vi "Log.vi"(0 "error handler in":refnum<class "TLB` Error Handler.lvclass">) -> (4 "error handler out":refnum<class "TLB` Error Handler.lvclass">, 15 "error out":errorcluster)   [LabVIEW 2015, in "TLB` Template.lvlib" / "TLB` Error Handler.lvclass"]
doc: "write capture errors to disk.\n\n<B>Input Parameters</B>\n\n<B>error handler in</B> dentifies your session. <B>Error Handler in</B> is obtained from the Open.vi of this class.\n\n<B>Output Parameters</B>\n\n<B>error handler out</B> identifies your session. <B>Error Handler out</B> is obtained from the Open.vi of this class.\n\n<B>error out</B> contains error information. This output provides standard error out functionality."
uses:
  TLB` Error Handler.lvclass
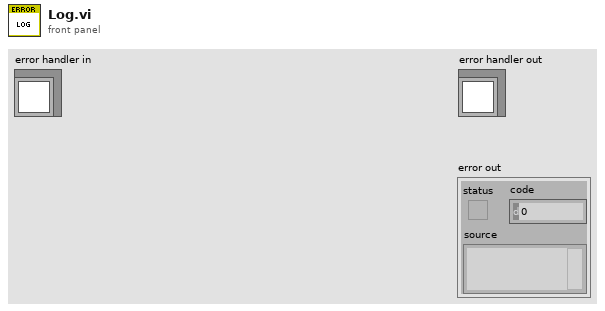
[diagram p1: front panel]
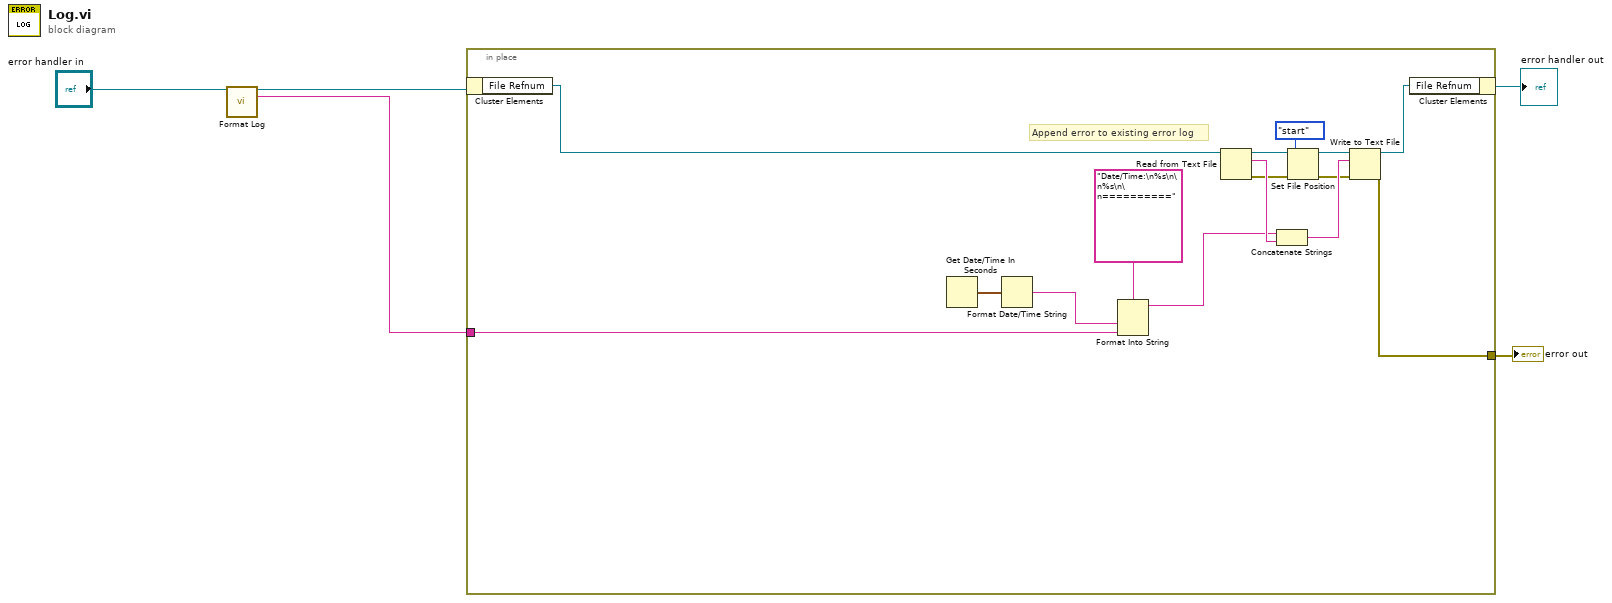
[diagram p0: block diagram]
diagram:
  n1 = call-dynamic "Format Log.vi"("error handler in"="error handler in") -> ("error handler out"=w2:refnum<class "TLB` Error Handler.lvclass">, "source text"=w1:string)  [unwired: 12 in, 1 out]
  n2 = in-place {
    in-place-border: [w19] -> w5
    in-place-border: w1 -> [w7]
    # "Append error to existing error log"
    n3 = in-place-cluster #1(w2) -> ("File Refnum"=w17:refnum<file>)
    n4 = Get Date/Time In Seconds() -> (seconds since 1Jan1904=w20:timestamp)
    n5 = Format Date/Time String(seconds (now)=w20) -> (date/time string=w9:string)  [unwired: 2 in]
    n6 = Format Into String(format string="Date/Time:\n%s\n\n%s\n\n==========", w9, w7) -> (resulting string=w6:string)  [unwired: 2 in, 1 out]
    n7 = Read from Text File(file (use dialog)=w17) -> (refnum out=w14:refnum<file>, text=w16:string, error out=w12:errorcluster)  [unwired: 3 in, 1 out]
    n8 = Concatenate Strings(w6, w16) -> (w15:string)
    n9 = Set File Position(refnum=w14, from (0:start)=enum16{"start", "end", "current"}."start", error in=w12) -> (refnum out=w13:refnum<file>, error out=w11:errorcluster)  [unwired: 1 in]
    n10 = Write to Text File(file (use dialog)=w13, text=w15, error in=w11) -> (refnum out=w18:refnum<file>, error out=w19:errorcluster)  [unwired: 1 in, 1 out]
    n11 = in-place-cluster #1("File Refnum"=w18) -> (→"error handler out":refnum<class "TLB` Error Handler.lvclass">)
  }
  "error out" <- w5
